vi "Close.vi"(8 "error in (no error)":errorcluster, 11 "reference in":refnum<class "Component_Template.lvclass">) -> (0 "error out":errorcluster, 3 "reference in":refnum<class "Component_Template.lvclass">)   [LabVIEW 2022 SP3, in "Component_Template.lvlib" / "Component_Template.lvclass"]
uses:
  Component_Template.lvclass
  Components/ViPER.lvlibp/ViPER.lvclass
  C:/Projects/Medulla/ViPER/ViPER_ProjectTemplates/ProjectTemplates/Source/Core/ViPER/Components/ViPER.lvlibp/ViPER.lvclass
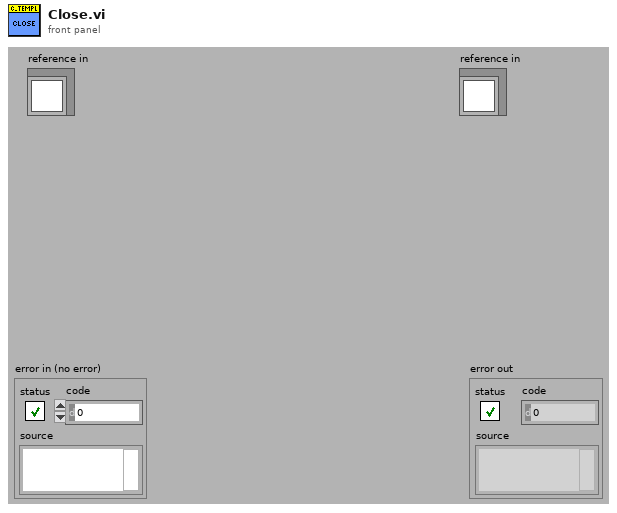
[diagram p1: front panel]
types:
  T1 = typedef "Component_Template.lvlib/Component_Template.lvclass/ObjectAttributes.ctl" = cluster{"Config":T2}
  T2 = typedef "Component_Template.lvlib/Component_Template.lvclass/Config.ctl" = cluster{"default":string}
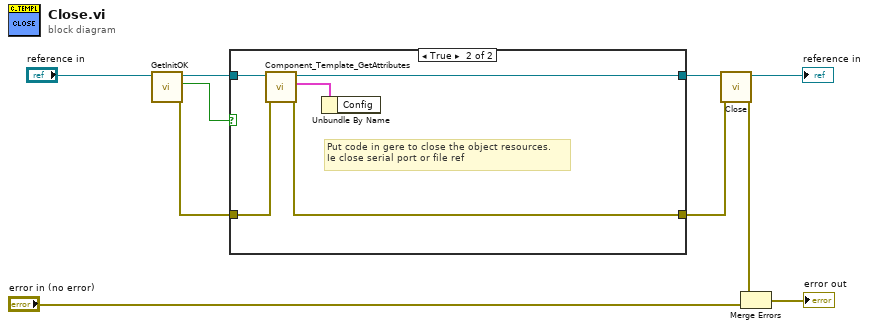
[diagram p0: block diagram]
diagram:
  n1 = call "GetInitOK.vi"("reference in"="reference in") -> ("error out"=w4:errorcluster, "init_ok"=w5:bool, "reference out"=w6:refnum<class "Component_Template.lvclass">)  [unwired: 8 in]
  n2 = case shown="True" w5 {
    tunnel: w4 -> [w12 w16]
    tunnel: [w12 w15] -> w7
    tunnel: w6 -> [w11 w17]
    tunnel: [w11 w13] -> w8
    frame False {
    }
    frame True {
      # "Put code in gere to close the object resources.\nIe close serial port or file ref"
      n3 = call "Component_Template_GetAttributes.vi"("error in (no error)"=w16, "reference in"=w17) -> ("error out"=w15:errorcluster, "Data"=w14:T1, "reference out"=w13:refnum<class "Component_Template.lvclass">)  [unwired: 6 in, 1 out]
      n4 = Unbundle By Name(w14) -> ()  [unwired: 1 out]
    }
  }
  n5 = call-parent "Close.vi"("error in (no error)"=w7, "reference in"=w8) -> ("error out"=w3:errorcluster, "reference out"=→"reference in":refnum<class "Component_Template.lvclass">)  [unwired: 8 in]
  n6 = Merge Errors(w3, "error in (no error)") -> (→"error out":errorcluster)
